vi "Table_AssertCellValue_Tests.vi"(8 "error in":errorcluster) -> (0 "error out":errorcluster)   [LabVIEW 2016, in "DronaTest.lvlib"]
uses:
  DronaTest.lvlib
  APIs/Stimulus/ControlValue/SetValueAuto.vi
  APIs/Assert/AssertControlValue/Controls/Table/AssertCellValue.vi
  <vilib>/addons/_JKI Toolkits/Caraya/classes/Assert/Assert Equal Value_Variant.vi
  <vilib>/addons/_JKI Toolkits/Caraya/classes/Test/Test.lvclass
  <vilib>/SLL Toolkit/SLL Debug/SLL Debug.lvlib
  Drona.lvlib
  <vilib>/addons/_JKI Toolkits/Caraya/classes/Assert/Assert.lvclass
  APIs/Get/GetControlRef/GetControlRef.lvlib
  APIs/Assert/AssertControlValue/Controls/Table/AssertTable.lvlib
  APIs/Stimulus/ControlValue/ControlValue.lvlib
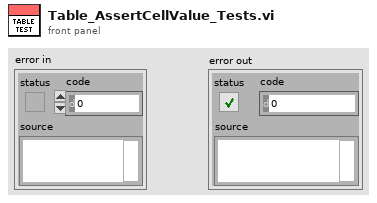
[diagram p1: front panel]
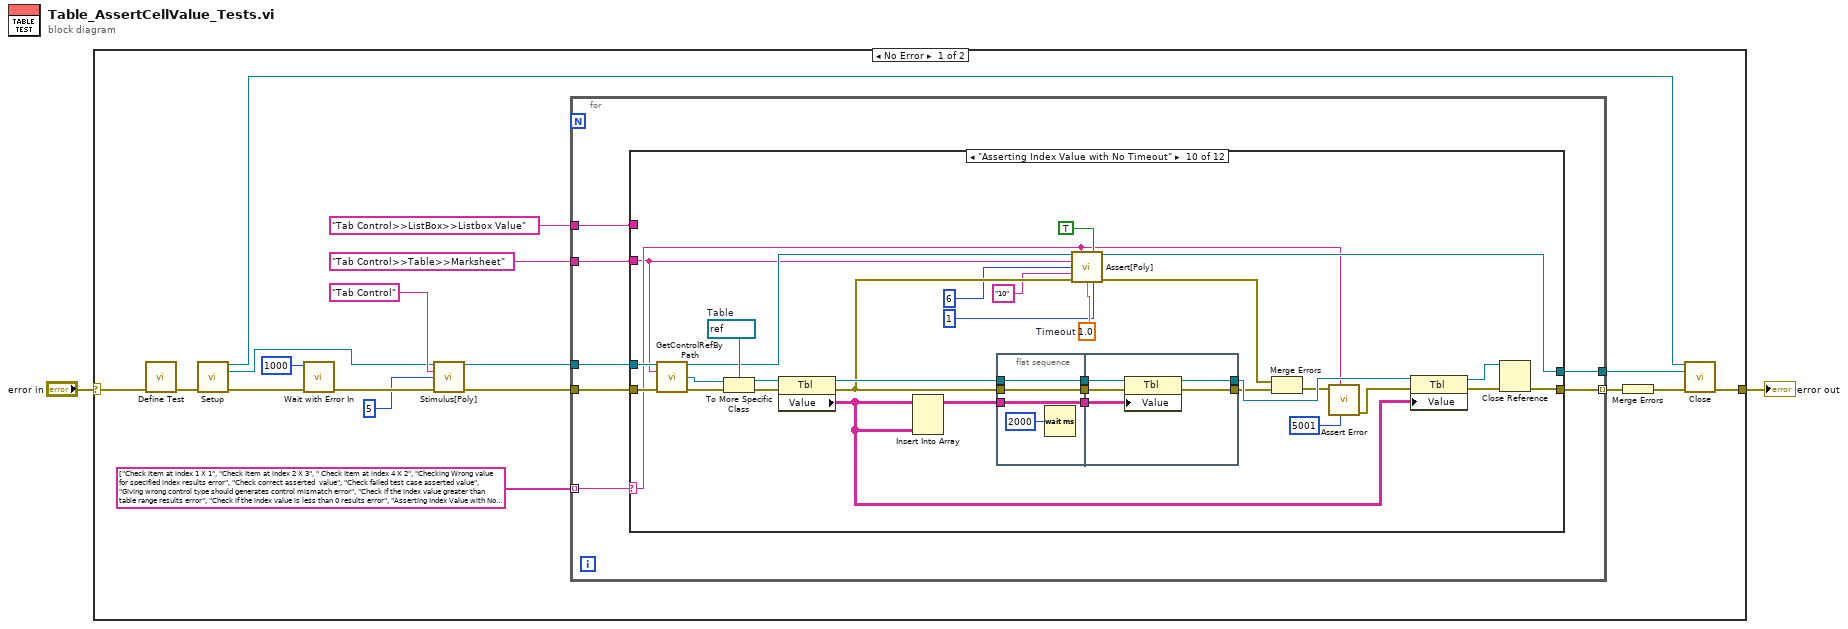
[diagram p0: block diagram]
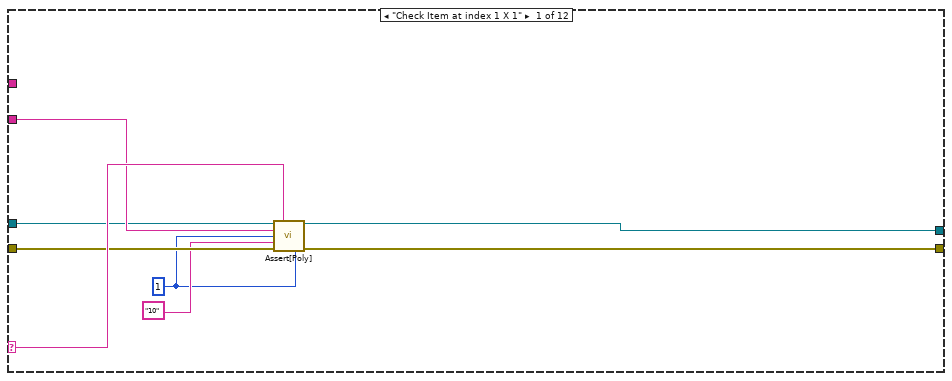
[diagram p2: hidden frame]
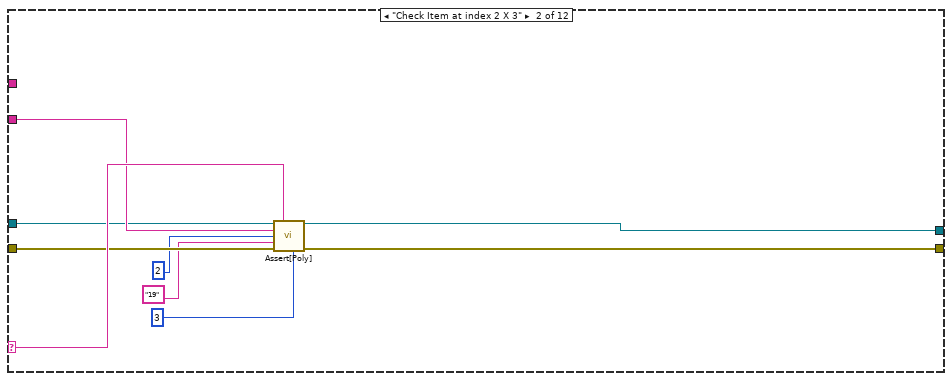
[diagram p3: hidden frame]
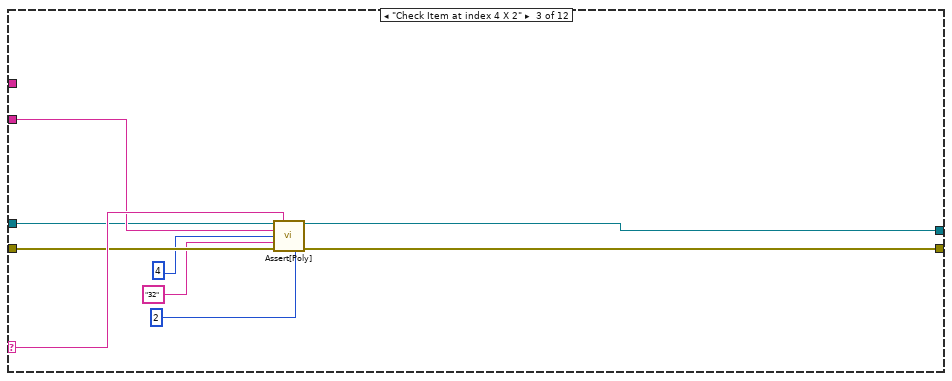
[diagram p4: hidden frame]
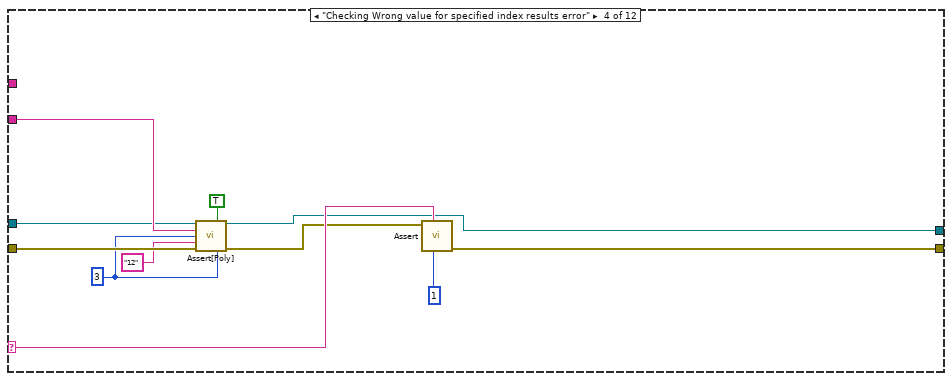
[diagram p5: hidden frame]
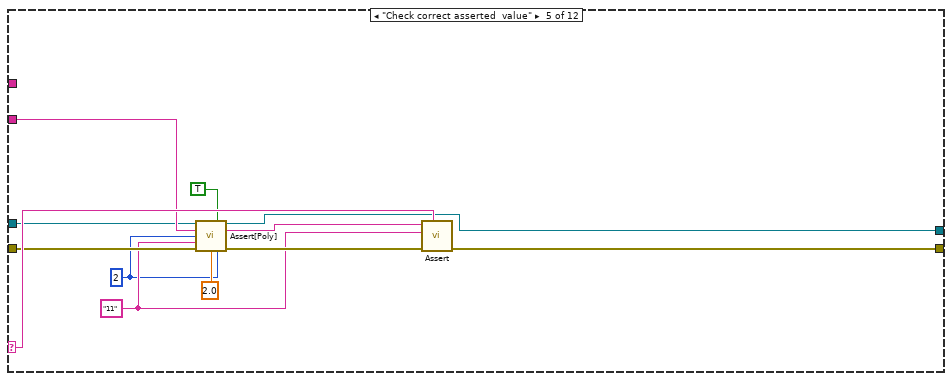
[diagram p6: hidden frame]
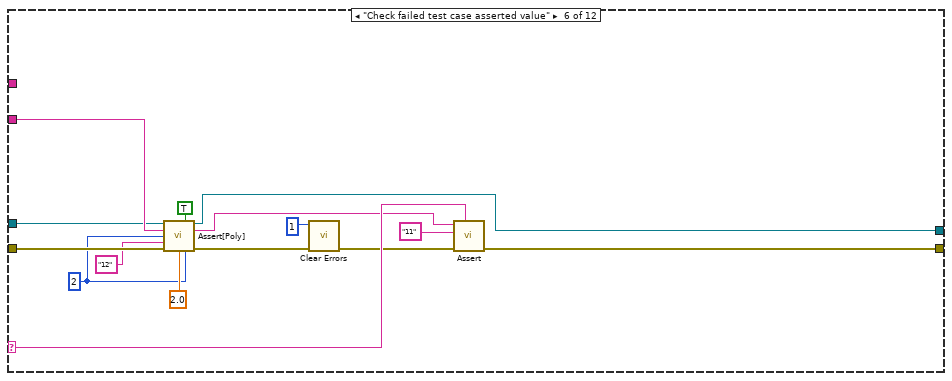
[diagram p7: hidden frame]
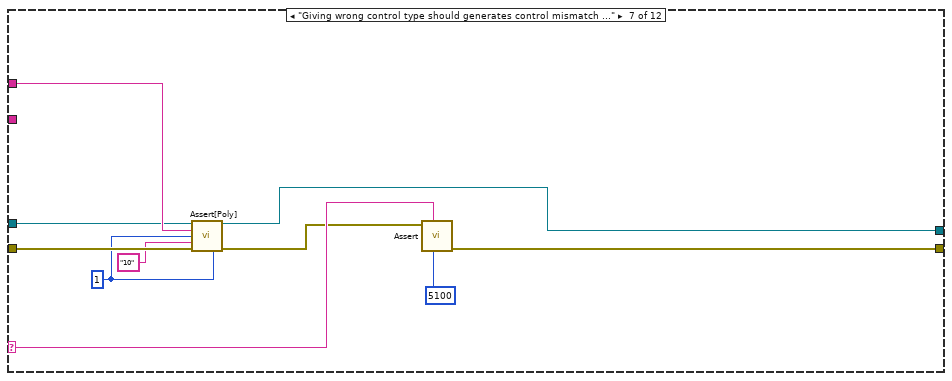
[diagram p8: hidden frame]
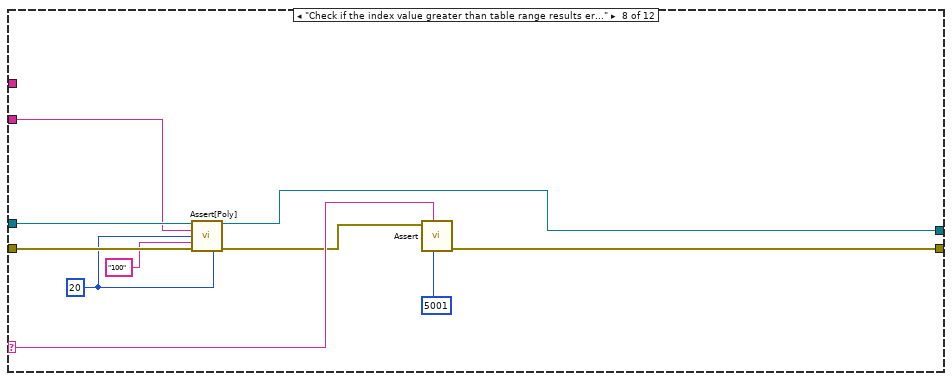
[diagram p9: hidden frame]
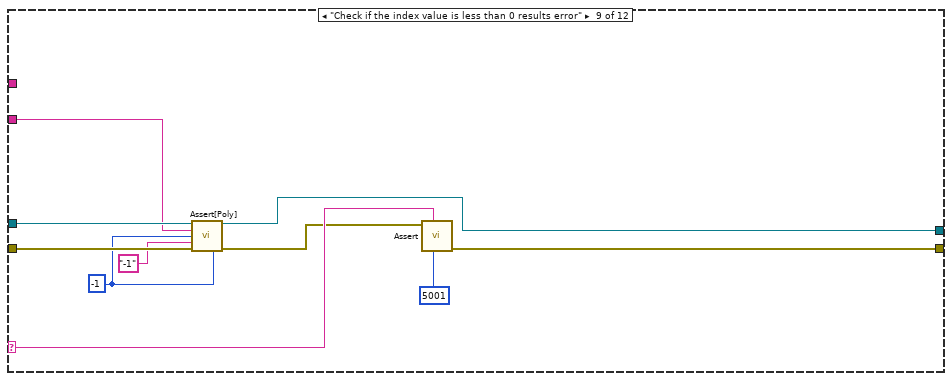
[diagram p10: hidden frame]
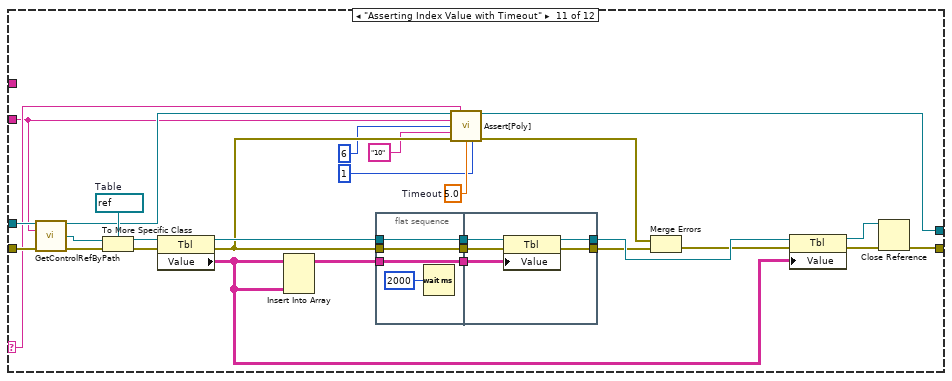
[diagram p11: hidden frame]
diagram:
  n1 = case shown="No Error" "error in" {
    selector: "error in" -> [w20 w203]
    tunnel: [w3 w203] -> w1
    frame No Error {
      n2 = call <vilib>:"Define Test.vi"("error in (no error)"=w20) -> ("error out"=w9:errorcluster)  [unwired: 9 in, 1 out]
      n3 = call "Setup.vi"("error in"=w9) -> ("Application Ref"=w5:refnum<vi>, "VI Reference Out"=w7:refnum<vi>, "error out"=w8:errorcluster)  [unwired: 12 in]
      n4 = call <vilib>:"Wait with Error In.vi"("error in (no error)"=w8, "milliseconds to wait"=u32 1000) -> ("error out"=w18:errorcluster)  [unwired: 9 in]
      n5 = call-poly "Stimulus[Poly].vi"("VI Reference In"=w7, "Control Path"="Tab Control", "Value (Signaling)"=5, "error in"=w18) -> ("VI Reference Out"=w14:refnum<vi>, "error out"=w17:errorcluster)  [unwired: 10 in]
      n6 = for {
        tunnel: w14 -> [w23]
        tunnel: "Tab Control>>Table>>Marksheet" ("Control Path") -> [w21]
        tunnel: "Tab Control>>ListBox>>Listbox Value" ("Control Path") -> [w22]
        tunnel: string[] ["Check Item at index 1 X 1", "Check Item at index 2 X 3", " Check Item at index 4 X 2", "Checking Wrong value for specified index results error", "Check correct asserted  value", "Check failed test case asserted value", "Giving wrong control type should generates control mismatch error", "Check if the index value greater than table range results error", "Check if the index value is less than 0 results error", "Asserting Index Value with No Timeout", "Asserting Index Value with Timeout"] -> [w27] mode=indexing
        tunnel: [w25] -> w4
        tunnel: w17 -> [w24]
        tunnel: [w26] -> w10 mode=indexing
        n7 = case shown="\"Asserting Index Value with No Timeout\"" w27 {
          selector: w27 -> [w33 w42 w51 w63 w75 w90 w100 w110 w120 w128 w181 _]
          tunnel: w24 -> [w31 w40 w49 w57 w71 w86 w95 w106 w116 w153 w191 w202]
          tunnel: w23 -> [w30 w39 w48 w56 w70 w85 w94 w105 w115 w151 w189 w201]
          tunnel: w21 -> [w32 w41 w50 w61 w74 w89 _ w103 w113 w122 w163 _]
          tunnel: w22 -> [_ _ _ _ _ _ w97 _ _ _ _ _]
          tunnel: [w35 w44 w53 w64 w76 w91 w101 w111 w121 w140 w177 w202] -> w26
          tunnel: [w34 w43 w52 w60 w73 w88 w96 w107 w117 w144 w182 w201] -> w25
          frame "Check Item at index 1 X 1" {
            w28 = 1 ("Item Index")
            n8 = call-poly "Assert[Poly].vi"("VI Reference In"=w30, "Test Label"=w33, "Control Path"=w32, "Row Index"=w28, "Item Value"="10", "Error In"=w31, "Column Index"=w28) -> ("VI Reference Out"=w34:refnum<vi>, "Error Out"=w35:errorcluster)  [unwired: 6 in, 1 out]
          }
          frame "Check Item at index 2 X 3" {
            n9 = call-poly "Assert[Poly].vi"("VI Reference In"=w39, "Test Label"=w42, "Control Path"=w41, "Row Index"=2 ("Item Index"), "Item Value"="19", "Error In"=w40, "Column Index"=3) -> ("VI Reference Out"=w43:refnum<vi>, "Error Out"=w44:errorcluster)  [unwired: 6 in, 1 out]
          }
          frame "Check Item at index 4 X 2" {
            n10 = call-poly "Assert[Poly].vi"("VI Reference In"=w48, "Test Label"=w51, "Control Path"=w50, "Row Index"=4 ("Item Index"), "Item Value"="32", "Error In"=w49, "Column Index"=2) -> ("VI Reference Out"=w52:refnum<vi>, "Error Out"=w53:errorcluster)  [unwired: 6 in, 1 out]
          }
          frame "Checking Wrong value for specified index results error" {
            w55 = 3 ("Item Index")
            n11 = call-poly "Assert[Poly].vi"("VI Reference In"=w56, "Assert Only? (F)"=TRUE, "Control Path"=w61, "Row Index"=w55, "Item Value"="12", "Error In"=w57, "Column Index"=w55) -> ("VI Reference Out"=w60:refnum<vi>, "Error Out"=w59:errorcluster)  [unwired: 6 in, 1 out]
            n12 = call-poly <vilib>:"Assert.vi"("error code (1)"=1, "Label"=w63, "Error?"=w59) -> ("error out"=w64:errorcluster)  [unwired: 7 in, 1 out]
          }
          frame "Check correct asserted  value" {
            w67 = "11" ("Item Value")
            w65 = 2 ("Item Index")
            n13 = call-poly "Assert[Poly].vi"("VI Reference In"=w70, "Assert Only? (F)"=TRUE, "Control Path"=w74, "Row Index"=w65, "Item Value"=w67, "Error In"=w71, "Timeout(5 sec)"=2.0, "Column Index"=w65) -> ("VI Reference Out"=w73:refnum<vi>, "Asserted Value"=w68:string, "Error Out"=w69:errorcluster)  [unwired: 5 in]
            n14 = call-poly <vilib>:"Assert.vi"("Label"=w75, "error in (no error)"=w69, "Y"=w67, "X"=w68) -> ("error out"=w76:errorcluster)  [unwired: 6 in, 1 out]
          }
          frame "Check failed test case asserted value" {
            w77 = 2 ("Item Index")
            n15 = call-poly "Assert[Poly].vi"("VI Reference In"=w85, "Assert Only? (F)"=TRUE, "Control Path"=w89, "Row Index"=w77, "Item Value"="12", "Error In"=w86, "Timeout(5 sec)"=2.0, "Column Index"=w77) -> ("VI Reference Out"=w88:refnum<vi>, "Asserted Value"=w83:string, "Error Out"=w84:errorcluster)  [unwired: 5 in]
            n16 = call <vilib>:"Clear Errors.vi"("error in (no error)"=w84, "specific error code to clear (0: all)"=1) -> ("error out"=w81:errorcluster)  [unwired: 4 in, 1 out]
            n17 = call-poly <vilib>:"Assert.vi"("Label"=w90, "error in (no error)"=w81, "Y"="11" ("Item Value"), "X"=w83) -> ("error out"=w91:errorcluster)  [unwired: 6 in, 1 out]
          }
          frame "Giving wrong control type should generates control mismatch error" {
            w92 = 1 ("Item Index")
            n18 = call-poly "Assert[Poly].vi"("VI Reference In"=w94, "Control Path"=w97, "Row Index"=w92, "Item Value"="10", "Error In"=w95, "Column Index"=w92) -> ("VI Reference Out"=w96:refnum<vi>, "Error Out"=w98:errorcluster)  [unwired: 7 in, 1 out]
            n19 = call-poly <vilib>:"Assert.vi"("error code (1)"=5100, "Label"=w100, "Error?"=w98) -> ("error out"=w101:errorcluster)  [unwired: 7 in, 1 out]
          }
          frame "Check if the index value greater than table range results error" {
            w102 = 20 ("Item Index")
            n20 = call-poly "Assert[Poly].vi"("VI Reference In"=w105, "Control Path"=w103, "Row Index"=w102, "Item Value"="100", "Error In"=w106, "Column Index"=w102) -> ("VI Reference Out"=w107:refnum<vi>, "Error Out"=w108:errorcluster)  [unwired: 7 in, 1 out]
            n21 = call-poly <vilib>:"Assert.vi"("error code (1)"=5001, "Label"=w110, "Error?"=w108) -> ("error out"=w111:errorcluster)  [unwired: 7 in, 1 out]
          }
          frame "Check if the index value is less than 0 results error" {
            w112 = -1 ("Item Index")
            n22 = call-poly "Assert[Poly].vi"("VI Reference In"=w115, "Control Path"=w113, "Row Index"=w112, "Item Value"="-1", "Error In"=w116, "Column Index"=w112) -> ("VI Reference Out"=w117:refnum<vi>, "Error Out"=w118:errorcluster)  [unwired: 7 in, 1 out]
            n23 = call-poly <vilib>:"Assert.vi"("error code (1)"=5001, "Label"=w120, "Error?"=w118) -> ("error out"=w121:errorcluster)  [unwired: 7 in, 1 out]
          }
          frame "Asserting Index Value with No Timeout" {
            w137 = 1.0  # Timeout
            w148 = refnum<vi> refnum  # Table
            n24 = call "GetControlRefByPath.vi"("VI Reference In"=w151, "Control Path"=w122, "error In"=w153) -> ("VI Reference Out"=w145:refnum<vi>, "Ctl Refnum"=w149:refnum<vi>, "error out"=w152:errorcluster)  [unwired: 10 in]
            n25 = To More Specific Class(target class=w148, reference=w149, error in=w152) -> (specific class reference=w147:refnum<vi>, error out=w150:errorcluster)
            n26 = property class="Tbl"(reference=w147, error in=w150) -> (reference out=w143:refnum<vi>, error out=w136:errorcluster, "Value"=w126:string[][])
            n27 = Insert Into Array(array=w126, new element=w126) -> (w146:string[][])  [unwired: 2 in]
            n28 = flat-sequence {
              tunnel: w136 -> [w155]
              tunnel: w143 -> [w156]
              tunnel: w146 -> [w157]
              tunnel: [w157] -> w134
              tunnel: [w156] -> w133
              tunnel: [w155] -> w132
              tunnel: [w160] -> w139
              tunnel: [w158] -> w135
              tunnel: w134 -> [w162]
              tunnel: w133 -> [w161]
              tunnel: w132 -> [w159]
              frame #0 {
                n29 = Wait (ms)(milliseconds to wait=u32 2000) -> ()  [unwired: 1 out]
              }
              frame #1 {
                n30 = property class="Tbl"(reference=w161, error in=w159, "Value"=w162) -> (reference out=w160:refnum<vi>, error out=w158:errorcluster)
              }
            }
            n31 = call-poly "Assert[Poly].vi"("VI Reference In"=w145, "Test Label"=w128, "Assert Only? (F)"=TRUE, "Control Path"=w122, "Row Index"=6, "Item Value"="10", "Error In"=w136, "Timeout(5 sec)"=w137, "Column Index"=1 ("Row Index")) -> ("VI Reference Out"=w144:refnum<vi>, "Error Out"=w142:errorcluster)  [unwired: 4 in, 1 out]
            n32 = Merge Errors(w142, w135) -> (w131:errorcluster)
            n33 = call <vilib>:"Assert Error.vi"("error code (1)"=5001, "Label"=w128, "Error?"=w131) -> ("error out"=w130:errorcluster)  [unwired: 7 in, 1 out]
            n34 = property class="Tbl"(reference=w139, error in=w130, "Value"=w126) -> (reference out=w138:refnum<vi>, error out=w141:errorcluster)
            n35 = Close Reference(reference=w138, error in (no error)=w141) -> (error out=w140:errorcluster)
          }
          frame "Asserting Index Value with Timeout" {
            w168 = 5.0  # Timeout
            w186 = refnum<vi> refnum  # Table
            n36 = call "GetControlRefByPath.vi"("VI Reference In"=w189, "Control Path"=w163, "error In"=w191) -> ("VI Reference Out"=w183:refnum<vi>, "Ctl Refnum"=w187:refnum<vi>, "error out"=w190:errorcluster)  [unwired: 10 in]
            n37 = To More Specific Class(target class=w186, reference=w187, error in=w190) -> (specific class reference=w185:refnum<vi>, error out=w188:errorcluster)
            n38 = property class="Tbl"(reference=w185, error in=w188) -> (reference out=w180:refnum<vi>, error out=w174:errorcluster, "Value"=w167:string[][])
            n39 = Insert Into Array(array=w167, new element=w167) -> (w184:string[][])  [unwired: 2 in]
            n40 = flat-sequence {
              tunnel: w174 -> [w193]
              tunnel: w180 -> [w194]
              tunnel: w184 -> [w195]
              tunnel: [w195] -> w171
              tunnel: [w194] -> w170
              tunnel: [w193] -> w169
              tunnel: [w198] -> w176
              tunnel: [w196] -> w172
              tunnel: w171 -> [w200]
              tunnel: w170 -> [w199]
              tunnel: w169 -> [w197]
              frame #0 {
                n41 = Wait (ms)(milliseconds to wait=u32 2000) -> ()  [unwired: 1 out]
              }
              frame #1 {
                n42 = property class="Tbl"(reference=w199, error in=w197, "Value"=w200) -> (reference out=w198:refnum<vi>, error out=w196:errorcluster)
              }
            }
            n43 = call-poly "Assert[Poly].vi"("VI Reference In"=w183, "Test Label"=w181, "Control Path"=w163, "Row Index"=6, "Item Value"="10", "Error In"=w174, "Timeout(5 sec)"=w168, "Column Index"=1 ("Row Index")) -> ("VI Reference Out"=w182:refnum<vi>, "Error Out"=w179:errorcluster)  [unwired: 5 in, 1 out]
            n44 = Merge Errors(w179, w172) -> (w173:errorcluster)
            n45 = property class="Tbl"(reference=w176, error in=w173, "Value"=w167) -> (reference out=w175:refnum<vi>, error out=w178:errorcluster)
            n46 = Close Reference(reference=w175, error in (no error)=w178) -> (error out=w177:errorcluster)
          }
          frame Default {
          }
        }
      }
      n47 = Merge Errors(w10) -> (w6:errorcluster)
      n48 = call "Close.vi"("Application Ref"=w5, "VI Reference"=w4, "error in"=w6) -> ("error out"=w3:errorcluster)  [unwired: 12 in]
    }
    frame Error {
    }
  }
  "error out" <- w1
